vi "dfd_Build Subband Filters from XML.vi"(6 "fs":dbl=1.0, 7 "Bank":enum16{"AnalysisBank", "SynthesisBank"}(ring), 8 "error in":errorcluster, 10 "content":string) -> (0 "error out":errorcluster, 2 "remain string":string, 3 "subband filters":T1[](array[typedef]) {"mMRate_SumWl" min=1 max=32 step=1; "mMRate_InputIwl" min=1 max=32 step=1; "mMRate_GainWl" min=1 max=32 step=1; "mMRate_OutputWl" min=1 max=32 step=1; "mMRate_InputWl" min=1 max=32 step=1; "mMRate_CoefWl" min=1 max=32 step=1; "mMRate_Mode" items=["Default"=-1, "No Rate Change"=0, "Interpolation"=1, "Decimation"=2, "Interpolated"=3, "Rational"=4]})   [LabVIEW 2017, in "NI_DigFilter_FilterBank.lvlib"]
uses:
  <vilib>/addons/Digital Filter Design/NI_DigFilter_FilterBank.lvlib
  <vilib>/addons/Digital Filter Design/_Objects.llb/DFD Multirate Filter Obj.ctl
  <vilib>/addons/Digital Filter Design/_Objects.llb/DFD Multirate Mode.ctl
  <vilib>/addons/Digital Filter Design/_Objects.llb/DFD Coef Norm Type.ctl
  <vilib>/addons/Digital Filter Design/_Objects.llb/DFD Round-off Mode.ctl
  <vilib>/addons/Digital Filter Design/_Objects.llb/DFD FXP MRate Multiply Mode.ctl
  <vilib>/addons/Digital Filter Design/NI_DigFilter_Process.lvlib
  <vilib>/addons/Digital Filter Design/NI_DigFilterLicensed.lvlib
panel:
  in  "subband filters":T1[](array[typedef]) {"mMRate_SumWl" min=1 max=32 step=1; "mMRate_InputIwl" min=1 max=32 step=1; "mMRate_GainWl" min=1 max=32 step=1; "mMRate_OutputWl" min=1 max=32 step=1; "mMRate_InputWl" min=1 max=32 step=1; "mMRate_CoefWl" min=1 max=32 step=1; "mMRate_Mode" items=["Default"=-1, "No Rate Change"=0, "Interpolation"=1, "Decimation"=2, "Interpolated"=3, "Rational"=4]}
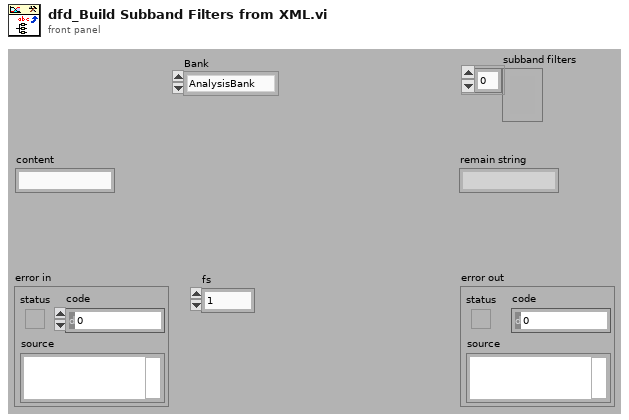
[diagram p1: front panel]
types:
  T1 = typedef "NI_DigFilterLicensed.lvlib/DFD Multirate Filter Obj.ctl" = cluster{"mMRate_Structure":enum16{"CIC", "FIR", "IIR", "Lattice"}, "mMRate_Mode":T2, "mMRate_Factor":i32, "mMRate_FIRParams":cluster{"mMRate_FIR_H":dbl[], "mMRate_FIR_IsNyquist?":bool, "mMRate_FIR_IsSymmetric?":bool}, "mMRate_CICParams":cluster{"mMRate_CIC_#Stage":i32, "mMRate_CIC_Lag":i32, "mMRate_CIC_Type":enum16{"Lowpass", "Highpass"}}, "mMRate_Order":i32, "mMRate_Version":string, "mMRate_Comments":string, "mMRate_RationalFactor":cluster{"mMRate_L":i32, "mMRate_M":i32}, "mMRate_Fs":dbl, "mMRate_Quantized?":bool, "mMRate_QFilterGain":dbl, "mMRate_CoefWl":i16, "mMRate_Scaling":cluster{"mMRate_ScaleByPowerOf2?":bool, "mMRate_ScaleType":T3}, "mMRate_InputWl":i16, "mMRate_OutputWl":i16, "mMRate_OutputMode":T4, "mMRate_MultMode":T5, "mMRate_BitPruning":bool, "mMRate_GainWl":i16, "mMRate_OutputFwl":i16, "mMRate_SumIwl":i16, "mMRate_InputIwl ":i16, "mMRate_SumWl":i16, "mMRate_CoefIwl":i16}
  T2 = typedef "NI_DigFilterLicensed.lvlib/DFD Multirate Mode.ctl" = i16
  T3 = typedef "NI_DigFilterLicensed.lvlib/DFD Coef Norm Type.ctl" = enum16{"No Norm", "Time Domain 1-Norm", "Time Domain 2-Norm", "Time Domain Inf-Norm"}
  T4 = typedef "NI_DigFilterLicensed.lvlib/DFD Round-off Mode.ctl" = enum16{"Nearest", "Truncation"}
  T5 = typedef "NI_DigFilterLicensed.lvlib/DFD FXP MRate Multiply Mode.ctl" = enum16{"Truncated", "Full"}
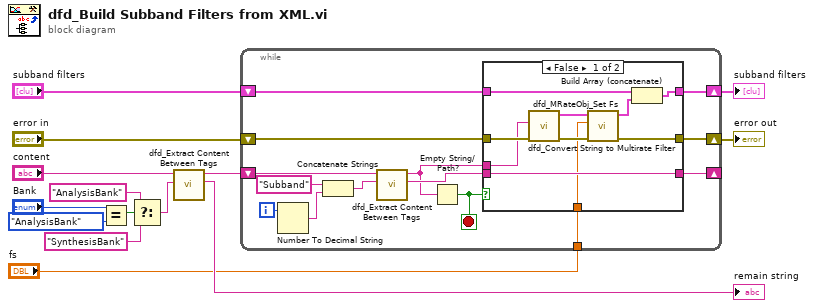
[diagram p0: block diagram]
diagram:
  n1 = Equal?(x="Bank", y=enum16{"AnalysisBank", "SynthesisBank"}."AnalysisBank") -> (x = y?=w5:bool)
  n2 = Select(t="AnalysisBank" ("string"), s=w5, f="SynthesisBank" ("string")) -> (s? t:f=w2:string)
  n3 = call <vilib>:"dfd_Extract Content Between Tags.vi"("element"=w2, "xml string with tag"="content") -> ("remaining string"=→"remain string":string, "content"=w10:string)  [unwired: 8 out]
  n4 = while {
    shift-right: [w27] -> w14
    shift-left: "error in" -> [w28]
    shift-right: [w19] -> _
    shift-left: w10 -> [w21]
    shift-right: [w16] -> w12
    shift-left: "subband filters" -> [w26]
    tunnel: "fs" -> [w15]
    i -> [w24]
    stop <- w17 stop-if-true
    n5 = Number To Decimal String(number=w24) -> (decimal integer string=w23:string)  [unwired: 1 out]
    n6 = Concatenate Strings("Subband" ("string"), w23) -> (w22:string)
    n7 = call <vilib>:"dfd_Extract Content Between Tags.vi"("element"=w22, "xml string with tag"=w21) -> ("remaining string"=w20:string, "content"=w18:string)  [unwired: 8 out]
    n8 = Empty String/Path?(string/path=w18) -> (empty?=w17:bool)
    n9 = case shown="False" w17 {
      tunnel: w28 -> [w37 w40]
      tunnel: [w31 w40] -> w27
      tunnel: w26 -> [w34 w38]
      tunnel: w18 -> [w36 _]
      tunnel: [w35 w39] -> w19
      tunnel: w20 -> [w35 w39]
      tunnel: [w33 w38] -> w16
      tunnel: w15 -> [w29 _]
      frame False {
        n10 = call <vilib>:"dfd_Convert String to Multirate Filter.vi"("error in (no error)"=w37, "xml string"=w36) -> ("error out"=w31:errorcluster, "multirate filter out"=w32:T1)  [unwired: 1 in, 7 out]
        n11 = call <vilib>:"dfd_MRateObj_Set Fs.vi"("fs"=w29, "multirate filter in"=w32) -> ("dup multirate filter"=w30:T1)  [unwired: 9 in]
        n12 = Build Array (concatenate)(w34, w30) -> (w33:T1[])
      }
      frame True {
      }
    }
  }
  "error out" <- w14
  "subband filters" <- w12
